vi "Read Device Address.vi"(8 "error in (no error)":errorcluster, 11 "ChannelConfig in":refnum<class "ChannelConfig.lvclass">) -> (0 "error out":errorcluster, 2 "Device Address":tag, 3 "ChannelConfig out":refnum<class "ChannelConfig.lvclass">)   [LabVIEW 2015, in "Channel.lvlib" / "ChannelConfig.lvclass"]
uses:
  ChannelConfig.lvclass
  ChannelConfig.lvclass/ChannelConfig.ctl
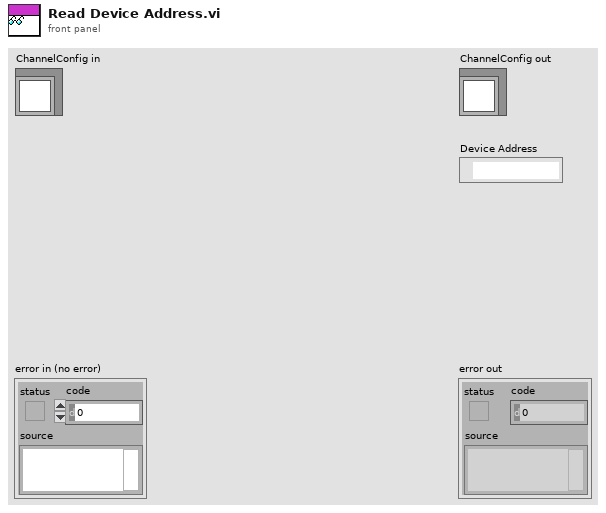
[diagram p1: front panel]
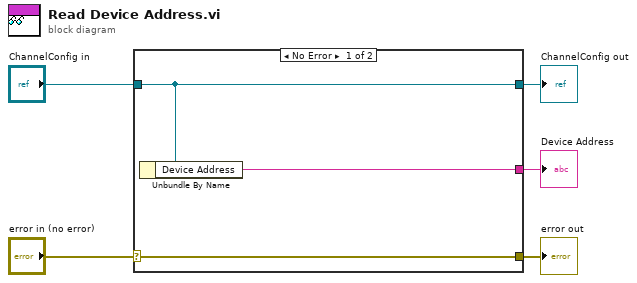
[diagram p0: block diagram]
diagram:
  n1 = case shown="No Error" "error in (no error)" {
    selector: "error in (no error)" -> [w8 w9]
    tunnel: [w8 w9] -> w4
    tunnel: [w7 w10] -> w2
    tunnel: "ChannelConfig in" -> [w7 w10]
    tunnel: [w6 _] -> w1
    frame No Error {
      n2 = Unbundle By Name(w7) -> ("Device Address"=w6:tag)
    }
    frame Error {
    }
  }
  "error out" <- w4
  "ChannelConfig out" <- w2
  "Device Address" <- w1
